vi "set log configure.vi"(8 "error in (no error)":errorcluster, 10 "log options":T1, 11 "set default (F)":bool) -> (0 "error out":errorcluster)   [LabVIEW 2024, in "atsj peakcan basic.lvlib"]
uses:
  atsj peakcan basic.lvlib
  log options.ctl
  parameter.ctl
  set parameter - i32.vi
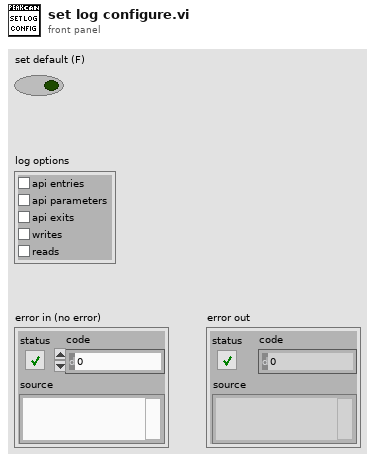
[diagram p1: front panel]
types:
  T1 = typedef "atsj peakcan basic.lvlib/log options.ctl" = cluster{"api entries":bool, "api parameters":bool, "api exits":bool, "writes":bool, "reads":bool}
  T2 = typedef "atsj peakcan basic.lvlib/parameter.ctl" = enum8{"DEVICE_ID", "5VOLTS_POWER", "RECEIVE_EVENT", "MESSAGE_FILTER", "API_VERSION", "CHANNEL_VERSION", "BUSOFF_AUTORESET", "LISTEN_ONLY", "LOG_LOCATION", "LOG_STATUS", "LOG_CONFIGURE", "LOG_TEXT", "CHANNEL_CONDITION", "HARDWARE_NAME", "RECEIVE_STATUS", "CONTROLLER_NUMBER", "TRACE_LOCATION", "TRACE_STATUS", "TRACE_SIZE", "TRACE_CONFIGURE", "CHANNEL_IDENTIFYING", "CHANNEL_FEATURES", "BITRATE_ADAPTING", "BITRATE_INFO", "BITRATE_INFO_FD", "BUSSPEED_NOMINAL", "BUSSPEED_DATA", "IP_ADDRESS", "LAN_SERVICE_STATUS", "ALLOW_STATUS_FRAMES", "ALLOW_RTR_FRAMES", "ALLOW_ERROR_FRAMES", "INTERFRAME_DELAY", "ACCEPTANCE_FILTER_11BIT", "ACCEPTANCE_FILTER_29BIT", "IO_DIGITAL_CONFIGURATION", "IO_DIGITAL_VALUE", "IO_DIGITAL_SET", "IO_DIGITAL_CLEAR", "IO_ANALOG_VALUE", "FIRMWARE_VERSION", "ATTACHED_CHANNELS_COUNT", "ATTACHED_CHANNELS", "ALLOW_ECHO_FRAMES", "DEVICE_PART_NUMBER", "HARD_RESET_STATUS", "LAN_CHANNEL_DIRECTION", "DEVICE_GUID"}
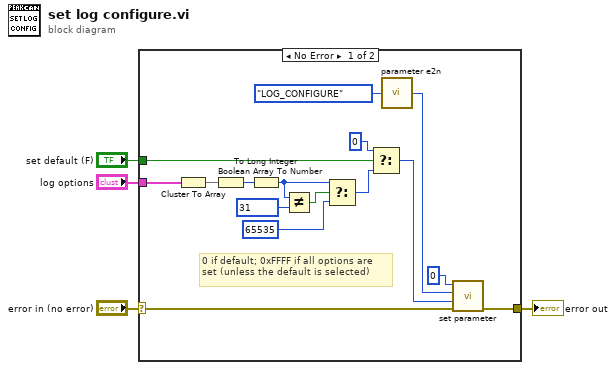
[diagram p0: block diagram]
diagram:
  n1 = case shown="No Error" "error in (no error)" {
    selector: "error in (no error)" -> [w20 w21]
    tunnel: [w19 w21] -> w3
    tunnel: "set default (F)" -> [w18 _]
    tunnel: "log options" -> [w16 _]
    frame No Error {
      # "0 if default; 0xFFFF if all options are set (unless the default is selected)"
      n2 = Cluster To Array(cluster=w16) -> (array=w15:bool[])
      n3 = Boolean Array To Number(Boolean array=w15) -> (number=w11:u32)
      n4 = To Long Integer(number=w11) -> (32bit integer=w9:i32)
      n5 = Not Equal?(x=w9, y=31) -> (x != y?=w12:bool)
      n6 = Select(t=w9, s=w12, f=65535) -> (s? t:f=w8:i32)
      n7 = Select(t=0, s=w18, f=w8) -> (s? t:f=w17:i32)
      n8 = call "parameter e2n.vi"("parameter"=parameter."LOG_CONFIGURE") -> ("number"=w5:u8)
      n9 = call-poly "set parameter.vi"("error in (no error)"=w20, "value"=w17, "parameter"=w5, "channel"=u16 0) -> ("error out"=w19:errorcluster)  [unwired: 7 in]
    }
    frame Error {
    }
  }
  "error out" <- w3
